vi "locate Single.vi"(8 "error in":errorcluster, 10 "name":string, 11 "data dictionary in":refnum<class "data dictionary.lvclass">) -> (0 "error out":errorcluster, 2 "index":i32, 3 "data dictionary out":refnum<class "data dictionary.lvclass">)   [LabVIEW 2013, in "tag bus.lvlib" / "data dictionary.lvclass"]
doc: "Locates a tag within the dictionary and provides its index within the associated data table."
uses:
  data dictionary.lvclass
  data dictionary.lvclass/data dictionary.ctl
  search/search string list.vi
  search/binary search.lvlib
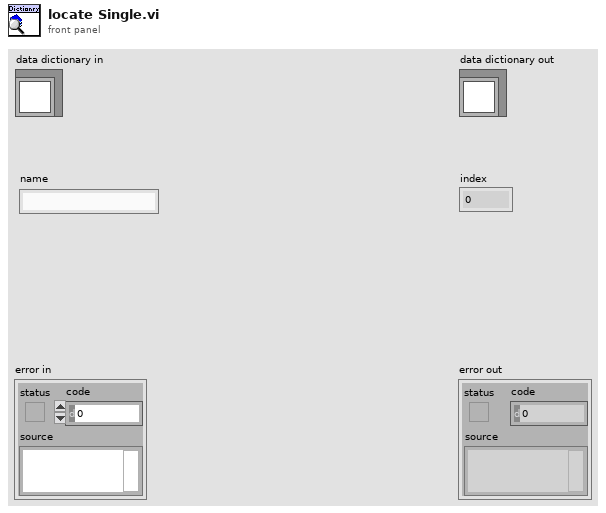
[diagram p1: front panel]
types:
  T1 = typedef "tag bus.lvlib/binary search.lvlib/sorted list.ctl" = cluster{"sorted strings":string[], "sorted indices":i32[]}
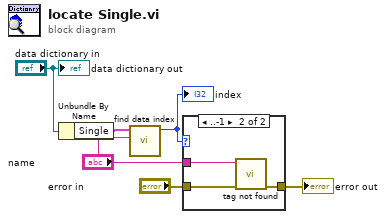
[diagram p0: block diagram]
diagram:
  n1 = Unbundle By Name("data dictionary in") -> ("Single"=w5:T1)
  n2 = call "find data index.vi"("string to locate"="name", "sorted list"=w5) -> ("index"=w4:i32)  [unwired: 9 in]
  "index" <- w4
  n3 = case shown="..-1" w4 {
    tunnel: [w7 w10] -> w2
    tunnel: "error in" -> [w7 w9]
    tunnel: "name" -> [_ w8]
    frame 0.. {
    }
    frame ..-1 {
      n4 = call "tag not found.vi"("error in"=w9, "name"=w8) -> ("error out"=w10:errorcluster)  [unwired: 9 in]
    }
  }
  "error out" <- w2
  "data dictionary out" <- "data dictionary in"
